vi "F CDF.vi"(9 "k2":i32=1, 10 "k1":i32=1, 11 "x":dbl=0.5) -> (0 "error":i32, 3 "cdf(x)":dbl=0.6065306597126334)   [LabVIEW 2017, in "NI_Gmath.lvlib"]
doc: "Computes the continuous cumulative distribution function (CDF), or the probability that the random variate X, where X describes the selected distribution type, has a value less than or equal to <B>x</B>. You must manually select the polymorphic instance to use."
uses:
  <vilib>/gmath/NI_Gmath.lvlib
  <vilib>/gmath/statdist.llb/st_error_code.ctl
  <vilib>/gmath/SpecialFunctions.llb/Incomplete Beta Function.vi
panel:
  # "F CDF"
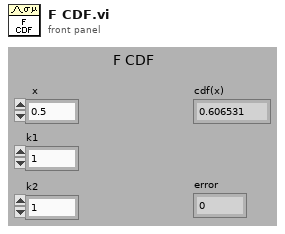
[diagram p1: front panel]
types:
  T1 = typedef "NI_Gmath.lvlib/st_error_code.ctl" = i32
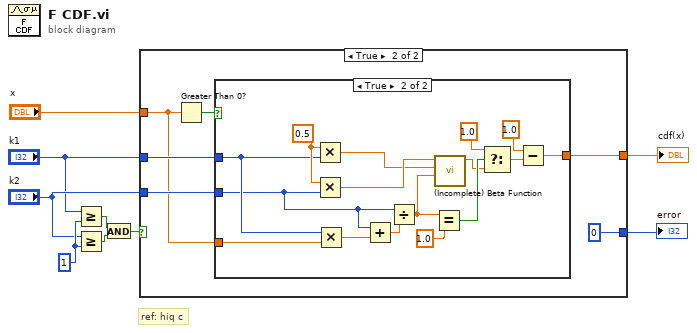
[diagram p0: block diagram]
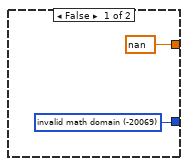
[diagram p2: hidden frame]
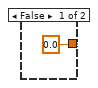
[diagram p3: hidden frame]
diagram:
  w3 = 1 ("y")
  # "ref: hiq c"
  n1 = Greater Or Equal?(x="k1", y=w3) -> (x >= y?=w4:bool)
  n2 = Greater Or Equal?(x="k2", y=w3) -> (x >= y?=w5:bool)
  n3 = And(x=w4, y=w5) -> (x .and. y?=w6:bool)
  n4 = case shown="True" w6 {
    tunnel: "k2" -> [_ w14]
    tunnel: [w10 0 ("invalid math domain")] -> w9
    tunnel: [nan w16] -> w8
    tunnel: "x" -> [_ w13]
    tunnel: "k1" -> [_ w15]
    frame False {
      w10 = T1 -20069 items=["invalid math domain"=-20069, "Fourier interpolation size m >= n"=-20070, "empty array"=-20003] ("stat interp error code")
    }
    frame True {
      n5 = Greater Than 0?(x=w13) -> (x > 0?=w12:bool)
      n6 = case shown="True" w12 {
        tunnel: [0.0 w25] -> w16
        tunnel: w13 -> [_ w32]
        tunnel: w15 -> [_ w33]
        tunnel: w14 -> [_ w28]
        frame False {
        }
        frame True {
          w34 = 0.5 ("x")
          n7 = Multiply(x=w34, y=w33) -> (x*y=w29:dbl)
          n8 = Multiply(x=w34, y=w28) -> (x*y=w30:dbl)
          n9 = Multiply(x=w33, y=w32) -> (x*y=w27:dbl)
          n10 = Add(x=w28, y=w27) -> (x+y=w31:dbl)
          n11 = Divide(x=w28, y=w31) -> (x/y=w19:dbl)
          n12 = Equal?(x=w19, y=1.0) -> (x = y?=w23:bool)
          n13 = call-poly <vilib>:"(Incomplete) Beta Function.vi"("a"=w19, "y"=w29, "x"=w30) -> ("b(x, y, a)"=w22:dbl)  [unwired: 8 in]
          n14 = Select(t=1.0, s=w23, f=w22) -> (s? t:f=w20:dbl)
          n15 = Subtract(x=1.0, y=w20) -> (x-y=w25:dbl)
        }
      }
    }
  }
  "cdf(x)" <- w8
  "error" <- w9
